vi "1WIRE_CONVERT_TEMP.vi"(7 "1-Wire DIO Pin":refnum<k21>="ConnectorA/DIO15", 8 "error in (no error)":errorcluster) -> (0 "error out":errorcluster, 3 "Convert Time (usec)":u32)   [LabVIEW 2014]
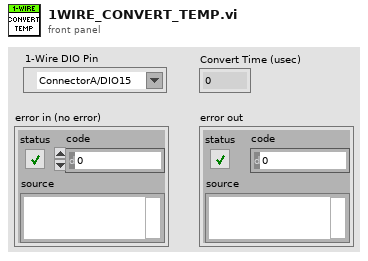
[diagram p1: front panel]
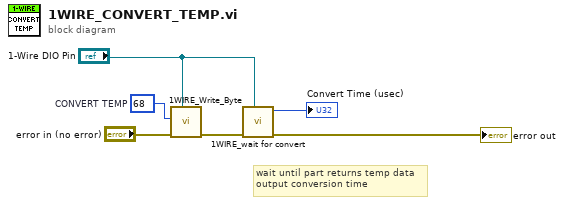
[diagram p0: block diagram]
diagram:
  w6 = u8 68  # CONVERT TEMP
  # "wait until part returns temp data\noutput conversion time"
  n1 = call "1WIRE_Write_Byte.vi"("1-Wire DIO Pin"="1-Wire DIO Pin", "error in"="error in (no error)", "Tx data"=w6) -> ("error out"=w4:errorcluster)  [unwired: 7 in, 1 out]
  n2 = call "1WIRE_wait for convert.vi"("1-Wire DIO Pin"="1-Wire DIO Pin", "error in"=w4) -> ("error out"=→"error out":errorcluster, "Convert Time (usec)"=→"Convert Time (usec)":u32)  [unwired: 8 in]
